vi "ShooterState.vi"() -> ()   [LabVIEW 2019]
panel:
  in  "Fire":bool
  in  "Speed":dbl
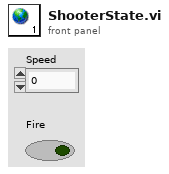
[diagram p1: front panel]
diagram:
